vi "strip_whitespace.vi"(10 "String in":string) -> (2 "String out":string)   [LabVIEW 2015, in "oskar_tools.lvlib"]
uses:
  oskar_tools.lvlib
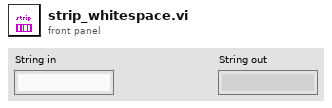
[diagram p1: front panel]
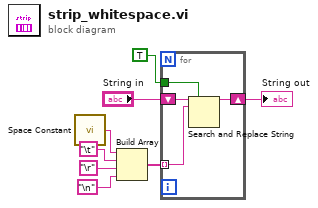
[diagram p0: block diagram]
diagram:
  n1 = call <vilib>:"Space Constant.vi"() -> ("String"=w8:string)
  n2 = Build Array(w8, "\t", "\r", "\n") -> (w2:string[])
  n3 = for {
    tunnel: TRUE ("replace all? (F)") -> [w11]
    shift-right: [w10] -> w3
    shift-left: "String in" -> [w12]
    tunnel: w2 -> [w9] mode=indexing
    n4 = Search and Replace String(replace all?=w11, input string=w12, search string=w9) -> (result string=w10:string)  [unwired: 5 in, 3 out]
  }
  "String out" <- w3
